vi "Lockin.DAQ.Clear.vi"(8 "error in (no error)":errorcluster, 11 "Lockin.DAQ in":refnum<class "Lockin.DAQ.lvclass">) -> (0 "error out":errorcluster, 3 "Lockin.DAQ out":refnum<class "Lockin.DAQ.lvclass">)   [LabVIEW 2016, in "Lockin.DAQ.lvclass"]
uses:
  Lockin.DAQ.lvclass
  Lockin.DAQ.lvclass/Lockin.DAQ.ctl
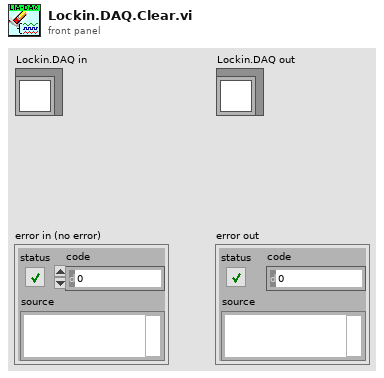
[diagram p1: front panel]
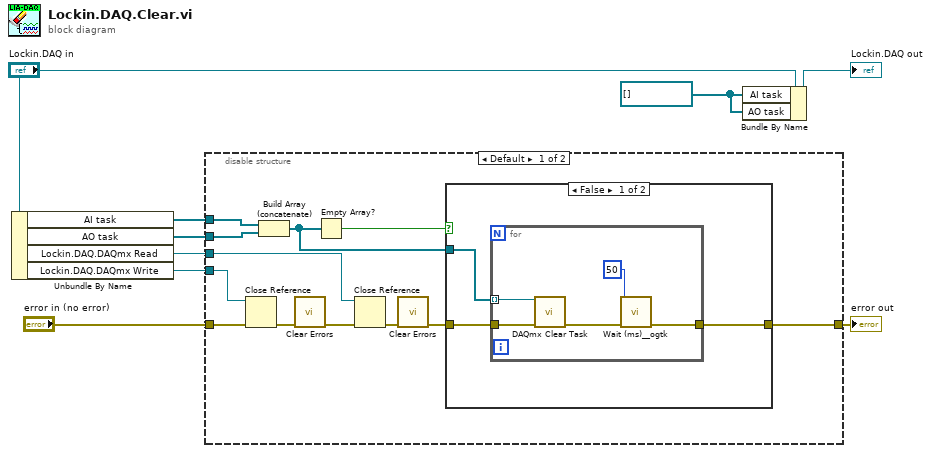
[diagram p0: block diagram]
diagram:
  w3 = refnum<k21>[] [] ("AI task")
  n1 = Unbundle By Name("Lockin.DAQ in") -> ("AI task"=w6:refnum<k21>[], "AO task"=w7:refnum<k21>[], "Lockin.DAQ.DAQmx Read"=w2:refnum<vi>, "Lockin.DAQ.DAQmx Write"=w1:refnum<vi>)
  n2 = disable-structure shown="Default" {
    disable-tunnel: "error in (no error)" -> [w16 _]
    disable-tunnel: [w19 _] -> w8
    disable-tunnel: w7 -> [w20 _]
    disable-tunnel: w6 -> [w21 _]
    disable-tunnel: w2 -> [w12 _]
    disable-tunnel: w1 -> [w13 _]
    frame condition #0 (active) {
      n3 = Close Reference(reference=w13, error in (no error)=w16) -> (error out=w15:errorcluster)
      n4 = Build Array (concatenate)(w21, w20) -> (w17:refnum<k21>[])
      n5 = call <vilib>:"Clear Errors.vi"("error in (no error)"=w15) -> ("error out"=w11:errorcluster)  [unwired: 5 in, 1 out]
      n6 = Empty Array?(array=w17) -> (empty?=w18:bool)
      n7 = Close Reference(reference=w12, error in (no error)=w11) -> (error out=w14:errorcluster)
      n8 = call <vilib>:"Clear Errors.vi"("error in (no error)"=w14) -> ("error out"=w10:errorcluster)  [unwired: 5 in, 1 out]
      n9 = case shown="False" w18 {
        tunnel: w10 -> [w22 w30]
        tunnel: w17 -> [w23 _]
        tunnel: [w24 w30] -> w19
        frame False {
          n10 = for {
            tunnel: w23 -> [w29] mode=indexing
            tunnel: w22 -> [w28]
            tunnel: [w25] -> w24
            n11 = call <vilib>:"DAQmx Clear Task.vi"("task in"=w29, "error in"=w28) -> ("error out"=w26:errorcluster)  [unwired: 13 in]
            n12 = call <userlib>:"Wait (ms)__ogtk.vi"("error in (no error)"=w26, "milliseconds to wait"=u32 50) -> ("error out"=w25:errorcluster)  [unwired: 8 in, 1 out]
          }
        }
        frame True {
        }
      }
    }
    frame condition #1 {
    }
  }
  "error out" <- w8
  n13 = Bundle By Name(cluster="Lockin.DAQ in", "AI task"=w3, "AO task"=w3) -> (→"Lockin.DAQ out":refnum<class "Lockin.DAQ.lvclass">)
